vi "OPCUA FinishTagGroup.vi"(8 "error in (no error)":errorcluster, 11 "reference":refnum<k24>) -> (0 "error out":errorcluster, 3 "reference 2":refnum<k24>)   [LabVIEW 2019]
uses:
  F:/src/HUTCDLSVN/Machine/CDL0100/TagEngine/LVOPCUA.NET/LVOPC.NETInterface/bin/Release/LVOPC.NETInterface.dll
  LVOPCUA.NET/LVOPC.NETInterface/bin/Release/LVOPC.NETInterface.dll
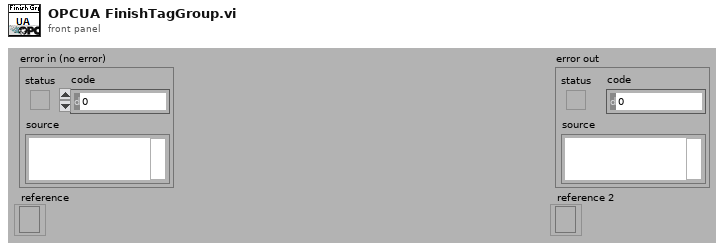
[diagram p1: front panel]
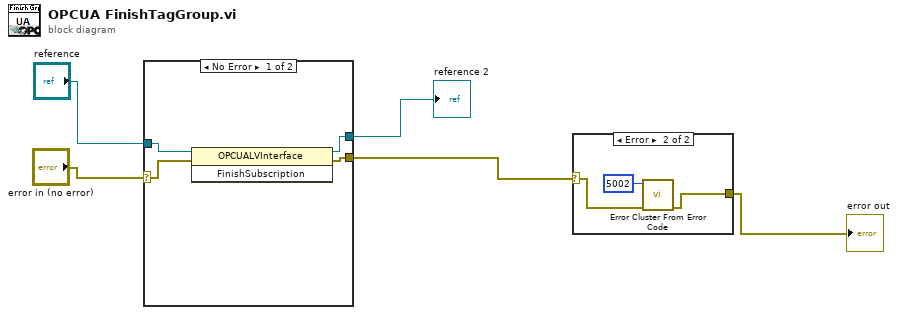
[diagram p0: block diagram]
diagram:
  n1 = case shown="No Error" "error in (no error)" {
    selector: "error in (no error)" -> [w8 w10]
    tunnel: "reference" -> [w9 w11]
    tunnel: [w7 w10] -> w2
    tunnel: [w6 w11] -> w1
    frame No Error {
      n2 = invoke class="OPCUALVInterface" method="FinishSubscription"(reference=w9, error in=w8) -> (reference out=w6:refnum<k24>, error out=w7:errorcluster)  [unwired: 1 in, 1 out]
    }
    frame Error {
    }
  }
  "reference 2" <- w1
  n3 = case shown="Error" w2 {
    selector: w2 -> [w12 w13]
    tunnel: [w12 w15] -> w5
    frame No Error {
    }
    frame Error {
      n4 = call <vilib>:"Error Cluster From Error Code.vi"("error in (no error)"=w13, "error code (0)"=5002) -> ("error out"=w15:errorcluster)  [unwired: 7 in]
    }
  }
  "error out" <- w5
